vi "MAT Stream Write Alloc Empty Data.vi"(6 "data type":T1, 7 "Matrix Name":string, 8 "error in (no error)":errorcluster, 9 "columns count":i32, 10 "rows count":i32, 11 "Ref Num":refnum<file>) -> (0 "error out":errorcluster, 1 "next var offset [B]":i64, 2 "data offset [B]":i64, 3 "Dup Ref Num":refnum<file>)   [LabVIEW 2018]
doc: "Matlab mat-v4 format lib: Prepares MAT file with header for one variable of given type. If the rows and columns counts are non-zero it will also set file size to the expected size of the variable matrix. It returns 'data offset [B]' which is start of the variable data area to be written and 'next var offset [B]' which is byte offset where next variable can be written."
uses:
  MAT Type Representation.ctl
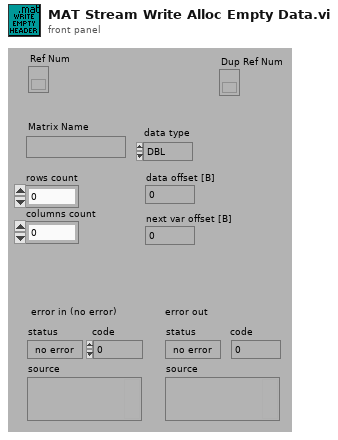
[diagram p1: front panel]
types:
  T1 = typedef "MAT Type Representation.ctl" = enum16{"DBL", "SGL", "I32", "I16", "U16", "U8", "CDB", "CSG", "STR"}
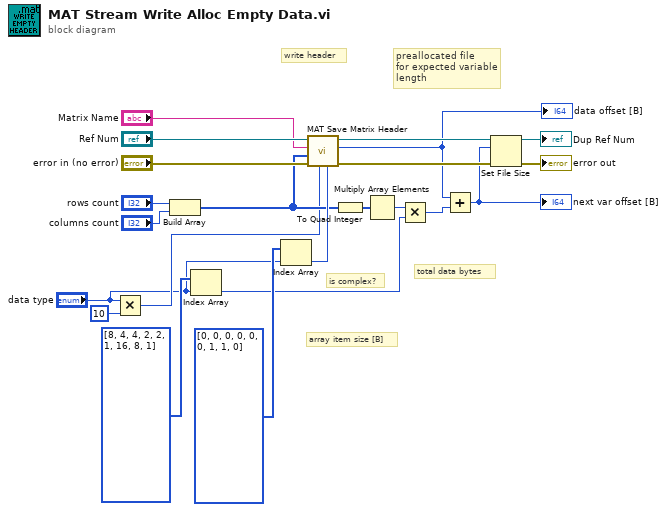
[diagram p0: block diagram]
diagram:
  # "write header"
  # "preallocated file\nfor expected variable\nlength"
  # "total data bytes"
  # "is complex?"
  # "array item size [B]"
  n1 = Multiply(x="data type", y=10) -> (x*y=w3:i32)
  n2 = Build Array("rows count", "columns count") -> (w12:i32[])
  n3 = Index Array(array=i64[] [8, 4, 4, 2, 2, 1, 16, 8, 1], index="data type") -> (element=w6:i64)
  n4 = Index Array(array=i32[] [0, 0, 0, 0, 0, 0, 1, 1, 0], index="data type") -> (element=w15:i32)
  n5 = call "MAT Save Matrix Header.vi"("Real/Complex (0-Real)"=w15, "Rep. Code"=w3, "error in (no error)"="error in (no error)", "Matrix Size"=w12, "Matrix Name"="Matrix Name", "Ref Num"="Ref Num") -> ("error out"=w14:errorcluster, "offset out"=w4:i64, "Dup Ref Num"=w13:refnum<file>)  [unwired: 3 in]
  "data offset [B]" <- w4
  n6 = To Quad Integer(1:w12) -> (0:w9:i64[])
  n7 = Multiply Array Elements(1:w9) -> (0:w7:i64)
  n8 = Multiply(x=w7, y=w6) -> (x*y=w5:i64)
  n9 = Add(x=w4, y=w5) -> (x+y=w8:i64)
  "next var offset [B]" <- w8
  n10 = Set File Size(4:w14, 6:w8, 7:w13) -> (0:→"error out":errorcluster, 3:→"Dup Ref Num":refnum<file>)
